vi "FlattenToXMLInternal.vi"(0 "Object in":refnum<class "OpenG_Value_Object.lvclass">, 9 "require data consistency (T)":bool=TRUE, 11 "error in (no error)":errorcluster, 12 "timeout in ms (-1)":i32=-1) -> (4 "Object out":refnum<class "OpenG_Value_Object.lvclass">, 6 "Object as XML":string, 8 "Before Child":string, 10 "After Child":string, 14 "time left":i32=-1, 15 "error out":errorcluster)   [LabVIEW 2015, in "OpenG_Value_Object.lvclass"]
doc: "Internal method to flatten object content to XML."
uses:
  <userlib>/_OpenG.lib/openg_object/openg_value_object.llb/OpenG_Value_Object.lvclass
  <userlib>/_OpenG.lib/openg_object/openg_object.llb/OpenG_Object.lvclass
panel:
  # "Please visit http://www.OpenG.org to learn about the\nOpen Source LabVIEW software movement.\n\nNOTICE -- YOU MUST LEAVE THIS NOTICE IN PLACE.  PER THE TERMS OF THE LICENSE BELOW, YOU MAY SUBLICENSE THIS SOFTWARE \nIN ANY WAY THAT DOES NOT CONFLICT WITH THIS LICENSE.\n\n### BSD License (http://www.opensource.org/licenses/bsd-license.php) Begin ###\n\nCopyright (c) 2007, Tomi Maila\nCopyright (c) 2007, Endevo AB\n\n\nAll rights reserved.\n\nRedistribution and use in source and binary forms, with or without modification, are permitted provided that the following conditions are met:\n\n    * Redistributions of source code must retain the above copyright notice, this list of conditions and the following disclaimer.\n    * Redistributions in binary form must reproduce the above copyright notice, this list of conditions and the following disclaimer in the \n       documentation and/or other materials provided with the distribution.\n    * Neither the name of Endevo AB nor the names of the contributors may be used to endorse or promote products derived\n       from this software without specific prior written permission.\n\nTHIS SOFTWARE IS PROVIDED BY THE COPYRIGHT HOLDERS AND CONTRIBUTORS \"AS IS\" AND ANY EXPRESS OR IMPLIED WARRANTIES, \nINCLUDING, BUT NOT LIMITED TO, THE IMPLIED WARRANTIES OF MERCHANTABILITY AND FITNESS FOR A PARTICULAR PURPOSE ARE \nDISCLAIMED. IN NO EVENT SHALL THE COPYRIGHT OWNER OR CONTRIBUTORS BE LIABLE FOR ANY DIRECT, INDIRECT, INCIDENTAL,\n SPECIAL, EXEMPLARY, OR CONSEQUENTIAL DAMAGES (INCLUDING, BUT NOT LIMITED TO, PROCUREMENT OF SUBSTITUTE GOODS OR \nSERVICES; LOSS OF USE, DATA, OR PROFITS; OR BUSINESS INTERRUPTION) HOWEVER CAUSED AND ON ANY THEORY OF LIABILITY, \nWHETHER IN CONTRACT, STRICT LIABILITY, OR TORT (INCLUDING NEGLIGENCE OR OTHERWISE) ARISING IN ANY WAY OUT OF THE USE \nOF THIS SOFTWARE, EVEN IF ADVISED OF THE POSSIBILITY OF SUCH DAMAGE.\n\n### BSD License End ###"
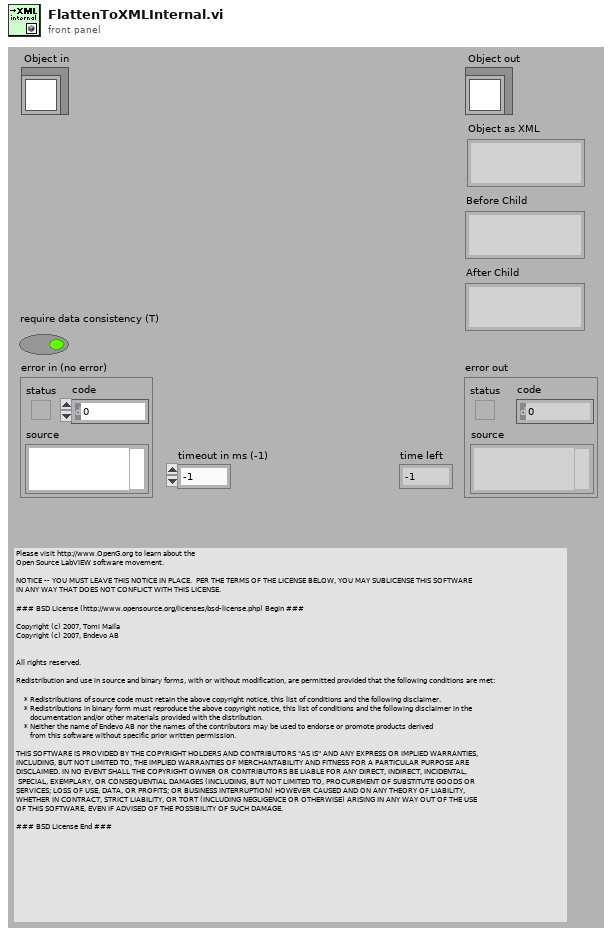
[diagram p1: front panel]
types:
  T1 = cluster{"Major":u16, "Minor":u16, "Fix":u16, "Build":u16}
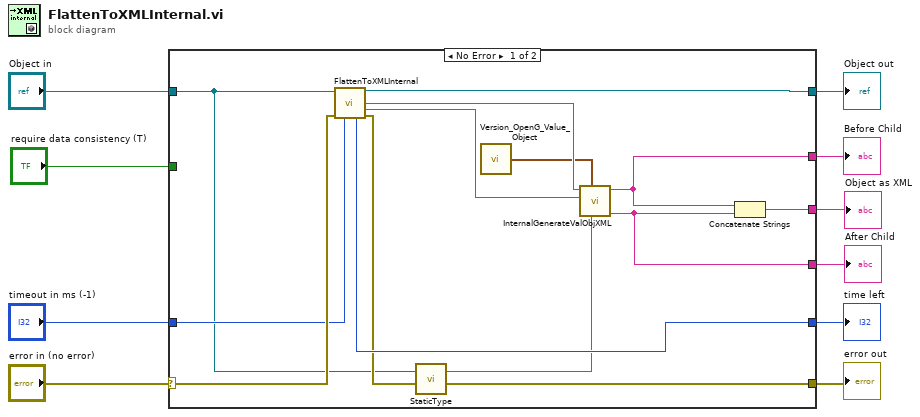
[diagram p0: block diagram]
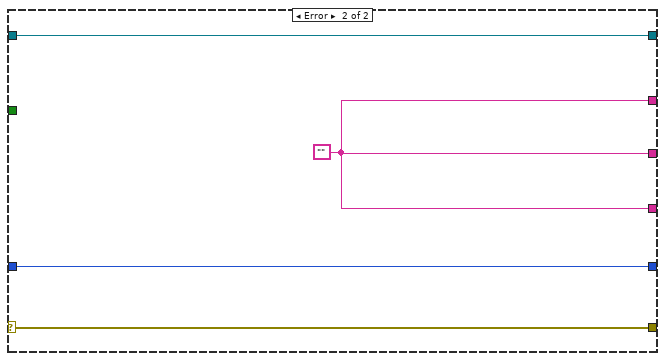
[diagram p2: hidden frame]
diagram:
  n1 = case shown="No Error" "error in (no error)" {
    selector: "error in (no error)" -> [w19 w26]
    tunnel: "Object in" -> [w11 w28]
    tunnel: [w24 w26] -> w9
    tunnel: [w23 w27] -> w8
    tunnel: [w22 w27] -> w7
    tunnel: [w21 w27] -> w6
    tunnel: [w20 w28] -> w5
    tunnel: "timeout in ms (-1)" -> [w18 w25]
    tunnel: "require data consistency (T)" -> [_ _]
    tunnel: [w17 w25] -> w1
    frame No Error {
      n2 = call-parent "FlattenToXMLInternal.vi"("Object in"=w11, "error in (no error)"=w19, "timeout in ms (-1)"=w18) -> ("Object out"=w20:refnum<class "OpenG_Value_Object.lvclass">, "Before Child"=w15:string, "After Child"=w14:string, "time left"=w17:i32, "error out"=w16:errorcluster)  [unwired: 7 in, 1 out]
      n3 = call <userlib>:"StaticType.vi"("error in (no error)"=w16, "Object in"=w11) -> ("error out"=w24:errorcluster, "static class name"=w13:string)  [unwired: 5 in]
      n4 = call <userlib>:"Version_OpenG_Value_Object.vi"() -> ("Version"=w12:T1)
      n5 = call <userlib>:"InternalGenerateValObjXML.vi"("static class name"=w13, "Class version"=w12, "Parent After Child"=w14, "Parent Before Child"=w15) -> ("After Child"=w21:string, "Before Child"=w22:string)  [unwired: 5 in, 1 out]
      n6 = Concatenate Strings(w22, w21) -> (w23:string)
    }
    frame Error {
      w27 = ""
    }
  }
  "error out" <- w9
  "Object out" <- w5
  "Object as XML" <- w8
  "Before Child" <- w7
  "After Child" <- w6
  "time left" <- w1
